vi "StartProgramsPLC.vi"(8 "error in (no error)":errorcluster, 9 "Номер банка программ":u16(ring) items=["0", "1", "2", "3", "4", "5", "6", "7"], 10 "Тип запроса":u16(ring) items=["Запуск программы", "Останов текущей программы"], 11 "StepMotor in":refnum<class "StepMotor.lvclass">) -> (0 "error out":errorcluster, 3 "StepMotor out":refnum<class "StepMotor.lvclass">)   [LabVIEW 2010, in "StepMotor.lvclass"]
doc: "Запуск программы в ПЛК двигателя СПШ"
uses:
  StepMotor.lvclass
  StepMotor.lvclass/StepMotor.ctl
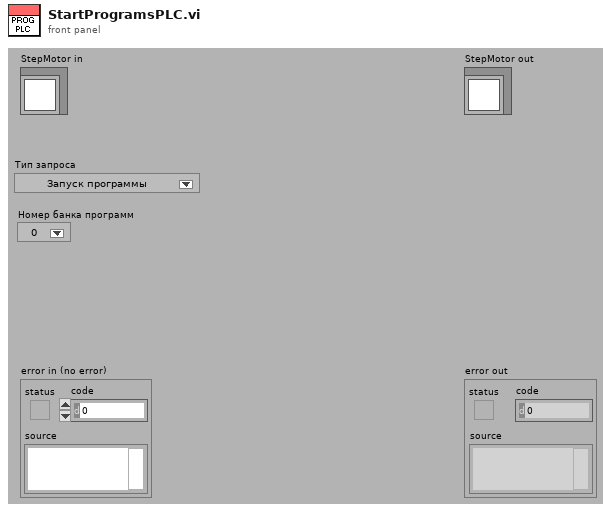
[diagram p1: front panel]
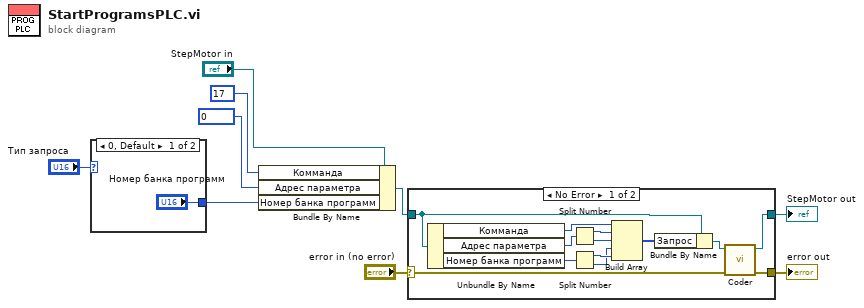
[diagram p0: block diagram]
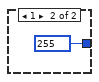
[diagram p2: hidden frame]
diagram:
  n1 = case shown="0, Default" "Тип запроса" {
    tunnel: ["Номер банка программ" u16 255 ("Адрес параметра")] -> w1
    frame 0, Default {
    }
    frame 1 {
    }
  }
  n2 = Bundle By Name(cluster="StepMotor in", "Комманда"=u8 17 ("Numeric"), "Адрес параметра"=u16 0, "Номер банка программ"=w1) -> (w5:refnum<class "StepMotor.lvclass">)
  n3 = case shown="No Error" "error in (no error)" {
    selector: "error in (no error)" -> [w20 w26]
    tunnel: [w19 w26] -> w8
    tunnel: [w21 w25] -> w7
    tunnel: w5 -> [w24 w25]
    frame No Error {
      n4 = Unbundle By Name(w24) -> ("Комманда"=w17:u8, "Адрес параметра"=w18:u16, "Номер банка программ"=w12:u16)
      n5 = Split Number(x=w18) -> (hi(x)=w16:u8, lo(x)=w15:u8)
      n6 = Split Number(x=w12) -> (hi(x)=w14:u8, lo(x)=w13:u8)
      n7 = Build Array(w17, w16, w15, w13, w14) -> (w23:u8[])
      n8 = Bundle By Name(cluster=w24, "Запрос"=w23) -> (w22:refnum<class "StepMotor.lvclass">)
      n9 = call "Coder.vi"("error in (no error)"=w20, "StepMotor in"=w22) -> ("error out"=w19:errorcluster, "StepMotor out"=w21:refnum<class "StepMotor.lvclass">)  [unwired: 8 in]
    }
    frame Error {
    }
  }
  "error out" <- w8
  "StepMotor out" <- w7
